vi "init.vi"(8 "error in (no error)":errorcluster, 11 "AlarmsTreeDisplayTC in":refnum<class "AlarmsTreeDisplayTC.lvclass">) -> (0 "error out":errorcluster, 2 "shared variables":refnum<k21>[](array[refnum])=["\\\\localhost\\M1PPubDataSV\\LoopTimeOutOfRange", "\\\\localhost\\M1PPubDataSV\\MsdLinPosOutOfRange", "\\\\localhost\\M1LPubDataSV\\LoopTimeOutOfRange", "\\\\localhost\\M1LPubDataSV\\MeasuredDeltaPressureHiIsTrue", "\\\\localhost\\M1LPubDataSV\\MeasuredTangentForceHiIsTrue"], 3 "AlarmsTreeDisplayTC out":refnum<class "AlarmsTreeDisplayTC.lvclass">)   [LabVIEW 2012, in "AlarmsTreeDisplayTC.lvclass"]
doc: "Initializes object."
uses:
  AlarmsTreeDisplayTC.lvclass
  C/Program Files (x86)/National Instruments/LabVIEW 2012/user.lib/Common/ComponentModel/ComponentModelDT/ConfigurationFileReaderDT/ConfigurationFileReaderDT.lvclass
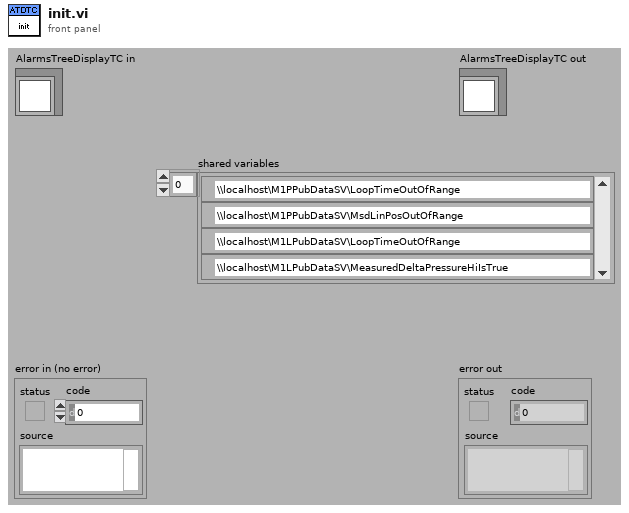
[diagram p1: front panel]
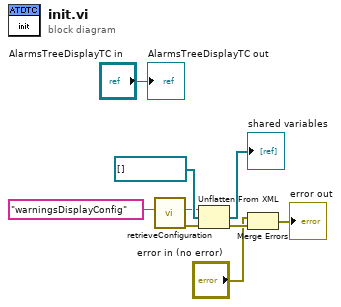
[diagram p0: block diagram]
diagram:
  n1 = call "retrieveConfiguration.vi"("dataName"="warningsDisplayConfig") -> ("error out"=w6:errorcluster, "dataValueFromFile"=w3:string)  [unwired: 8 in, 1 out]
  n2 = Unflatten From XML(xml string=w3, type=refnum<k21>[] [] ("warningsDisplayConfig"), error in (no error)=w6) -> (value=→"shared variables":refnum<k21>[], error out=w4:errorcluster)
  n3 = Merge Errors("error in (no error)", w4) -> (→"error out":errorcluster)
  "AlarmsTreeDisplayTC out" <- "AlarmsTreeDisplayTC in"
